vi "AudioTest.Parse Sealed Mic Result.vi"(6 "ErrorCode":i32=-5000, 7 "Measurement Name":string, 8 "error in":errorcluster, 9 "SoundCheckData Name(s)":string="LEFT_MIC_SENSITIVITY", 10 "Seq Name":string="UTAH_MP_SEQUENCE_SEALED_MIC 2019-01-23", 11 "Result Folder":path) -> (0 "error out":errorcluster, 1 "Found":bool, 2 "Mic Level":dbl, 3 "Meas":T1[](array[typedef]) {"Status" items=["LOG", "PASS", "FAIL", "ERROR"]})   [LabVIEW 2018]
uses:
  Common/Utils/Results/Result.Measurement Item.ctl
  Common/Utils/Results/Result.Measurement and Attribute Item Status.ctl
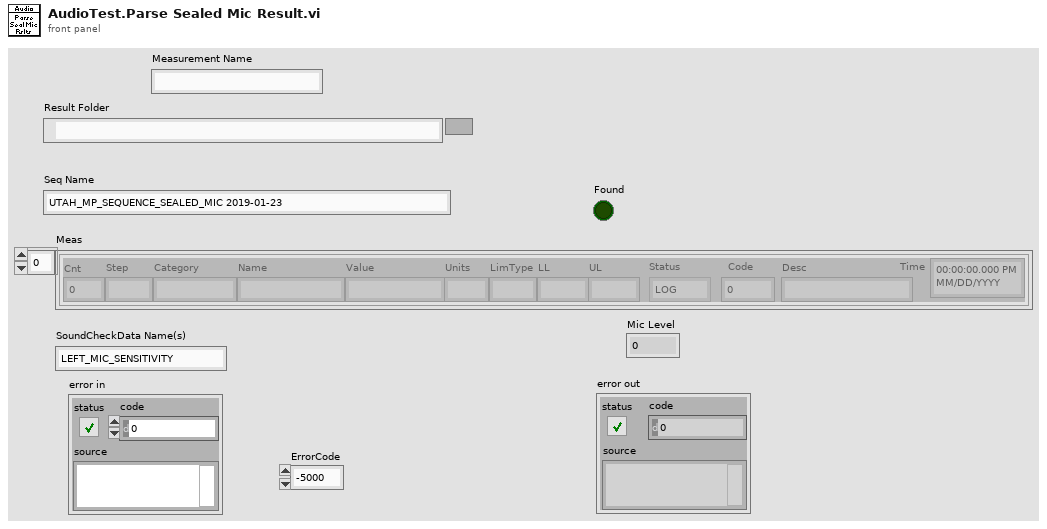
[diagram p1: front panel]
types:
  T1 = typedef "Result.Measurement Item.ctl" = cluster{"Cnt":i32, "Step":string, "Category":string, "Name":string, "Value":string, "Units":string, "LimType":string, "LL":string, "UL":string, "Status":T2, "Code":i32, "Desc":string, "Time":timestamp}
  T2 = typedef "Result.Measurement and Attribute Item Status.ctl" = i32
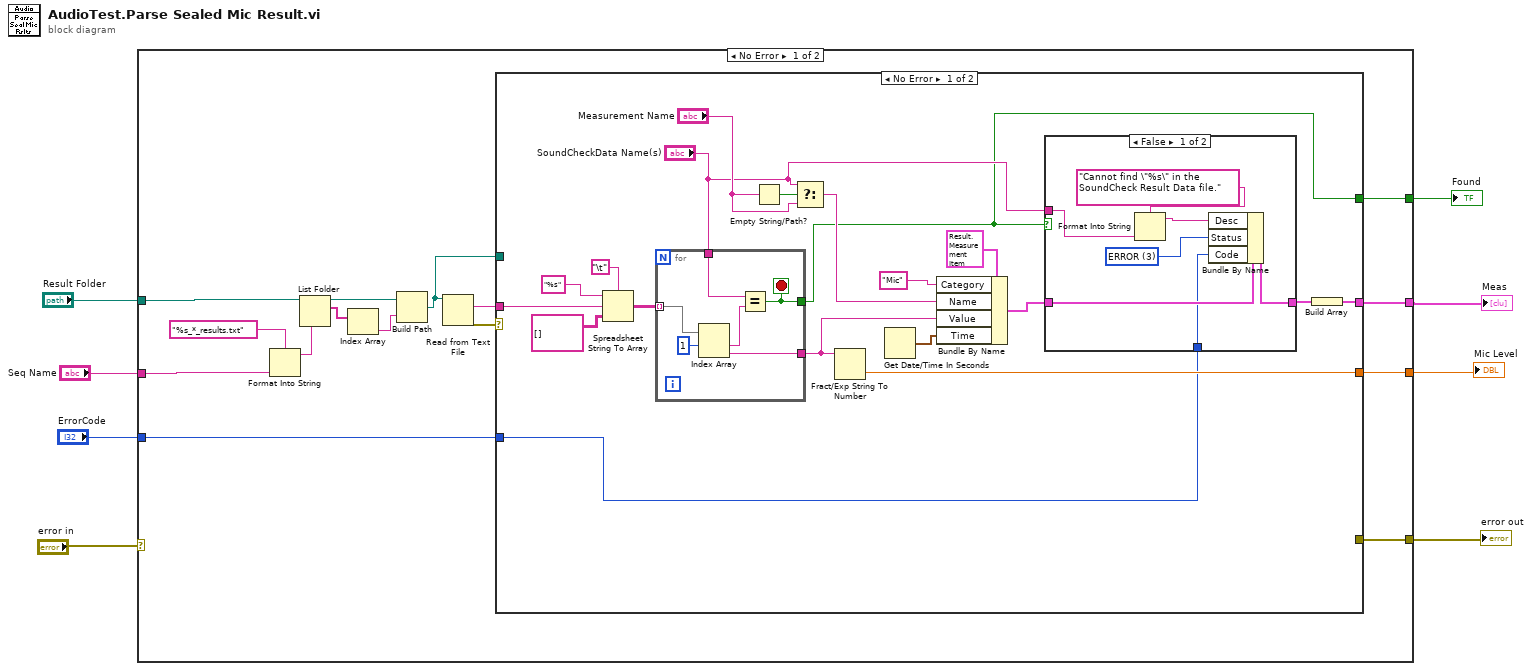
[diagram p0: block diagram]
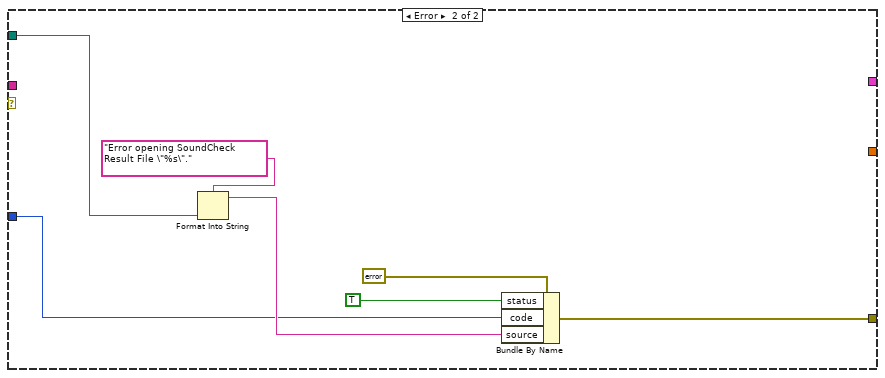
[diagram p3: hidden frame]
diagram:
  n1 = case shown="No Error" "error in" {
    tunnel: "Seq Name" -> [w21 _]
    tunnel: "Result Folder" -> [w20 _]
    tunnel: "ErrorCode" -> [w14 _]
    tunnel: [w12 _] -> w4
    tunnel: [w11 _] -> w3
    tunnel: [w10 _] -> w2
    tunnel: [w9 _] -> w1
    frame No Error {
      n2 = Format Into String(format string="%s_*_results.txt", w21) -> (resulting string=w19:string)  [unwired: 2 in, 1 out]
      n3 = List Folder(path=w20, pattern=w19) -> (path out=w17:path, filenames=w18:string[])  [unwired: 2 in, 2 out]
      n4 = Index Array(array=w18) -> (element=w23:string)  [unwired: 1 in]
      n5 = Build Path(base path=w17, name or relative path=w23) -> (appended path=w13:path)
      n6 = Read from Text File(file (use dialog)=w13) -> (text=w16:string, error out=w15:errorcluster)  [unwired: 3 in, 2 out]
      n7 = case shown="No Error" w15 {
        tunnel: w16 -> [w40 _]
        tunnel: w14 -> [w28 w58]
        tunnel: w13 -> [_ w62]
        tunnel: [_ w57] -> w12
        tunnel: [w37 _] -> w11
        tunnel: [w26 _] -> w10
        tunnel: [w24 _] -> w9
        frame No Error {
          n8 = Spreadsheet String To Array(delimiter (Tab)="\t", format string="%s", spreadsheet string=w40, array type (2D Dbl)=string[][] []) -> (array=w38:string[][])
          n9 = for {
            tunnel: w38 -> [w56] mode=indexing
            tunnel: [w55] -> w24
            tunnel: [w54] -> w34
            tunnel: "SoundCheckData Name(s)" -> [w53]
            stop <- w55 stop-if-true
            n10 = Index Array(array=w56, index #1=1 ("index")) -> (element #1=w52:string, element #2=w54:string)  [unwired: 1 in]
            n11 = Equal?(x=w53, y=w52) -> (x = y?=w55:bool)
          }
          n12 = Empty String/Path?(string/path="Measurement Name") -> (empty?=w32:bool)
          n13 = Select(t="SoundCheckData Name(s)", s=w32, f="Measurement Name") -> (s? t:f=w30:string)
          n14 = Fract/Exp String To Number(string=w34) -> (number=w37:dbl)  [unwired: 3 in, 1 out]
          n15 = Get Date/Time In Seconds() -> (seconds since 1Jan1904=w29:timestamp)
          n16 = Bundle By Name(cluster=T1 {"Cnt"=0, "Step"="", "Category"="", "Name"="", "Value"="", "Units"="", "LimType"="", "LL"="", "UL"="", "Status"=0, "Code"=0, "Desc"="", "Time"=timestamp(0 s since 1904-01-01)} ("Meas"), "Category"="Mic", "Name"=w30, "Value"=w34, "Time"=w29) -> (w33:T1)
          n17 = case shown="False" w24 {
            tunnel: w33 -> [w49 w50]
            tunnel: [w48 w50] -> w27
            tunnel: "SoundCheckData Name(s)" -> [w46 _]
            tunnel: w28 -> [w43 _]
            frame False {
              w44 = T2 3 items=["LOG", "PASS", "FAIL", "ERROR"] ("Status")
              n18 = Format Into String(format string="Cannot find \"%s\" in the SoundCheck Result Data file.", w46) -> (resulting string=w45:string)  [unwired: 2 in, 1 out]
              n19 = Bundle By Name(cluster=w49, "Desc"=w45, "Status"=w44, "Code"=w43) -> (w48:T1)
            }
            frame True {
            }
          }
          n20 = Build Array(w27) -> (w26:T1[])
        }
        frame Error {
          n21 = Format Into String(format string="Error opening SoundCheck Result File \"%s\".", w62) -> (resulting string=w59:string)  [unwired: 2 in, 1 out]
          n22 = Bundle By Name(cluster=errorcluster {"status"=TRUE, "code"=0, "source"=""} ("error constant"), "status"=TRUE, "code"=w58, "source"=w59) -> (w57:errorcluster)
        }
      }
    }
    frame Error {
    }
  }
  "Mic Level" <- w3
  "error out" <- w4
  "Meas" <- w2
  "Found" <- w1
